vi "Write vi reference.vi"(8 "error in (no error)":errorcluster caption="entrée d'erreur (pas d'erreur)", 10 "vi reference":refnum<vi>, 11 "Detector en entrée":refnum<class "Detector.lvclass">) -> (0 "error out":errorcluster caption="sortie d'erreur", 3 "Detector en sortie":refnum<class "Detector.lvclass">)   [LabVIEW 2019, in "Detector.lvclass"]
uses:
  Detector.lvclass
  Detector.lvclass/Detector.ctl
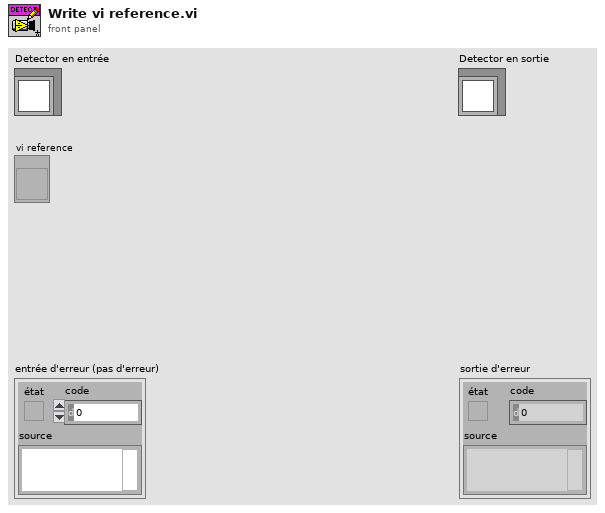
[diagram p1: front panel]
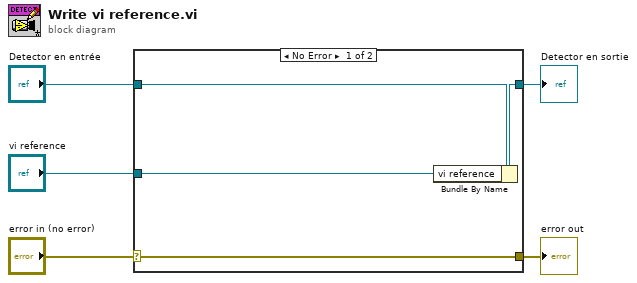
[diagram p0: block diagram]
diagram:
  n1 = case shown="No Error" "error in (no error)" {
    selector: "error in (no error)" -> [w9 w10]
    tunnel: [w9 w10] -> w4
    tunnel: [w7 w11] -> w2
    tunnel: "Detector en entrée" -> [w8 w11]
    tunnel: "vi reference" -> [w6 _]
    frame No Error {
      n2 = Bundle By Name(cluster=w8, "vi reference"=w6) -> (w7:refnum<class "Detector.lvclass">)
    }
    frame Error {
    }
  }
  "error out" <- w4
  "Detector en sortie" <- w2
